vi "dvp Vi Get Ae Target Descr.vi"(6 "piDefault":i32, 7 "piMax":i32, 9 "piMin":i32, 10 "piStep":i32, 11 "handle":u32) -> (1 "piMin out":i32, 2 "piStep out":i32, 3 "function return":u32(ring), 4 "piDefault out":i32, 5 "piMax out":i32)   [LabVIEW 2018, in "LabViewDVPCamera.lvlib"]
doc: "LabviewDvp2Api dvpStatus dvpViGetAeTargetDescr(\n dvpHandle handle,\n dvpInt32 *piStep,\n dvpInt32 *piMin,\n dvpInt32 *piMax,\n dvpInt32 *piDefault\n );"
uses:
  LabViewDVPCamera.lvlib
  LabViewDVPCamera/LabViewDVPCamera.dll
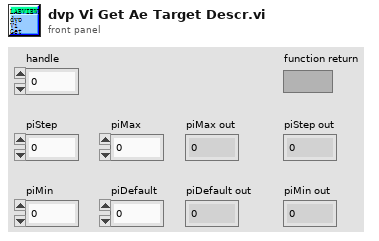
[diagram p1: front panel]
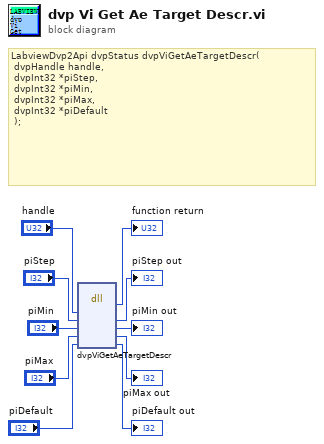
[diagram p0: block diagram]
diagram:
  # "LabviewDvp2Api dvpStatus dvpViGetAeTargetDescr(\n\tdvpHandle handle,\n\tdvpInt32 *piStep,\n\tdvpInt32 *piMin,\n\tdvpInt32 *piMax,\n\tdvpInt32 *piDefault\n\t);"
  n1 = dll-call lib="C:/Program Files (x86)/DVP2 Labview cn 64/Sample/LabViewDVPCamera/LabViewDVPCamera.*" fn="dvpViGetAeTargetDescr"("handle"="handle", "piStep"="piStep", "piMin"="piMin", "piMax"="piMax", "piDefault"="piDefault") -> (→"function return":u32, "piStep"=→"piStep out":i32, "piMin"=→"piMin out":i32, "piMax"=→"piMax out":i32, "piDefault"=→"piDefault out":i32)  [unwired: 4 in, 2 out]
